vi "IMUdata.vi"() -> ()   [LabVIEW 2016]
uses:
  Project Custom Controls/IMU Data Cluster.ctl
  <vilib>/myRIO/Common/Instrument Driver Framework/myRIO v1.0/UART/vis/myRIO v1.0 Close UART.vi
  <vilib>/Instr/_visa.llb/VISA Configure Serial Port (Instr).vi
  <vilib>/myRIO/Common/Instrument Driver Framework/Utilities/vis/FPGA Ref Manager.vi
  <vilib>/myRIO/Common/Instrument Driver Framework/myRIO v1.0/myRIO v1.0 Reset FPGA.vi
  <vilib>/myRIO/Common/Instrument Driver Framework/myRIO v1.0/IRQ/vis/myRIO v1.0 IRQ Info FGV.vi
  <vilib>/myRIO/Common/Instrument Driver Framework/myRIO v1.0/IRQ/vis/myRIO v1.0 Timer IRQ Info FGV.vi
  <vilib>/myRIO/Common/Instrument Driver Framework/myRIO v1.0/IRQ/vis/myRIO v1.0 ISR Agent.vi
  <vilib>/myRIO/Instrument Drivers/Utilities/Utilities.lvlib
panel:
  out "Waveform Chart":cluster{"Yaw":dbl, "Pitch":dbl, "Roll":dbl}(graph)
  in  "Stop":bool
  out "error out":errorcluster
  out "IMU Data Cluster":T1
  out "IMU Text":string
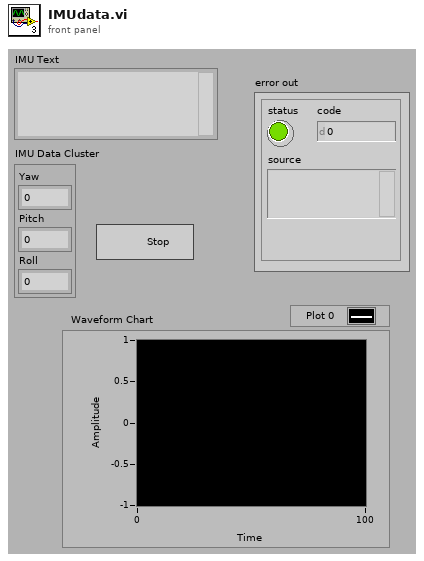
[diagram p1: front panel]
types:
  T1 = typedef "IMU Data Cluster.ctl" = cluster{"Yaw":dbl, "Pitch":dbl, "Roll":dbl}
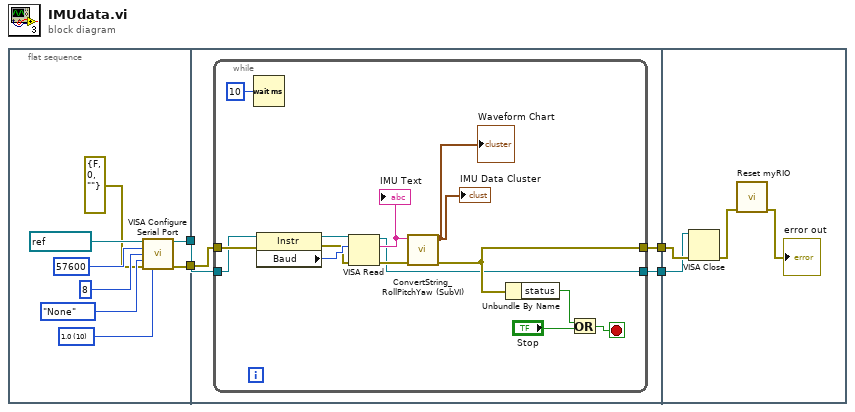
[diagram p0: block diagram]
diagram:
  n1 = flat-sequence {
    tunnel: [w6] -> w4
    tunnel: [w7] -> w3
    tunnel: w4 -> [w14]
    tunnel: w3 -> [w13]
    tunnel: [w16] -> w2
    tunnel: [w15] -> w1
    tunnel: w2 -> [w34]
    tunnel: w1 -> [w33]
    frame #0 {
      w11 = u16 10 items=["1.0"=10, "1.5"=15, "2.0"=20] ("stop bits (10: 1 bit)")
      n2 = call-poly "VISA Configure Serial Port"("VISA resource name"=refnum<visa-resource-name> "ASRL2::INSTR", "baud rate (9600)"=u32 57600, "data bits (8)"=u16 8, "parity (0:none)"=enum16{"None", "Odd", "Even", "Mark", "Space"}."None", "error in (no error)"=errorcluster {"status"=FALSE, "code"=0, "source"=""}, "stop bits (10: 1 bit)"=w11) -> ("VISA resource name out"=w7:refnum<visa-resource-name>, "error out"=w6:errorcluster)  [unwired: 8 in]
    }
    frame #1 {
      n3 = while {
        tunnel: w14 -> [w22]
        tunnel: [w28] -> w16
        tunnel: w13 -> [w21]
        tunnel: [w19] -> w15
        stop <- w30 stop-if-true
        n4 = Wait (ms)(milliseconds to wait=u32 10) -> ()  [unwired: 1 out]
        n5 = property class="Instr"(reference=w21, error in=w22) -> (reference out=w25:refnum<visa-resource-name>, error out=w26:errorcluster, "Baud"=w27:u32)
        n6 = VISA Read(VISA resource name=w25, byte count=w27, error in (no error)=w26) -> (VISA resource name out=w19:refnum<visa-resource-name>, read buffer=w23:string, error out=w24:errorcluster)  [unwired: 1 out]
        "IMU Text" <- w23
        n7 = call "ConvertString_RollPitchYaw (SubVI).vi"("error in (no error)"=w24, "IMU String Data"=w23) -> ("error out"=w28:errorcluster, "IMU Data Cluster"=→"IMU Data Cluster" →"Waveform Chart":T1)  [unwired: 8 in]
        n8 = Unbundle By Name(w28) -> ("status"=w29:bool)
        n9 = Or(x=w29, y="Stop") -> (x .or. y?=w30:bool)
      }
    }
    frame #2 {
      n10 = VISA Close(VISA resource name=w33, error in (no error)=w34) -> (error out=w32:errorcluster)
      n11 = call <vilib>:"Reset myRIO.vi"("error in (no error)"=w32) -> ("error out"=→"error out":errorcluster)  [unwired: 10 in]
    }
  }
